vi "encoders_periodic.vi"() -> ()   [LabVIEW 2020]
uses:
  <vilib>/Rock Robotics/WPI/ThirdParty/Phoenix-LabVIEW/CANCoder/Get/CTRE_Phoenix_CANcoder_GetSensorData.vi
  Swerve/swerve_globals.vi
  <vilib>/Rock Robotics/WPI/ThirdParty/Phoenix-LabVIEW/CANCoder/Set/CTRE_Phoenix_CANcoder_SetPositionToAbsolute.vi
  TitanLib/Lib/TitanLib.lvlib
panel:
  in  "Set Mag Offset?":bool
  in  "Encoder Offsets":dbl[](array[numeric])
  out "Encoders":dbl[](array[numeric])
  in  "Reset Encoders?":bool
  # "Pos"
  # "Abs"
  # "Pos"
  # "Abs"
  # "Pos"
  # "Abs"
  # "Pos"
  # "Abs"
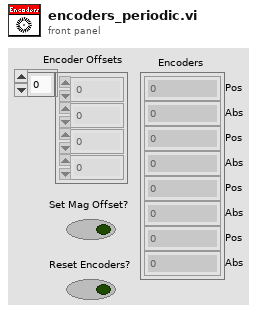
[diagram p1: front panel]
types:
  T1 = typedef "CTRE_Phoenix_CANcoder_DeviceRef.ctl" = cluster{"DeviceStatus":errorcluster, "Device Number":u8, "Handle":u64, "UsageFrame":u32, "Library Path":path}
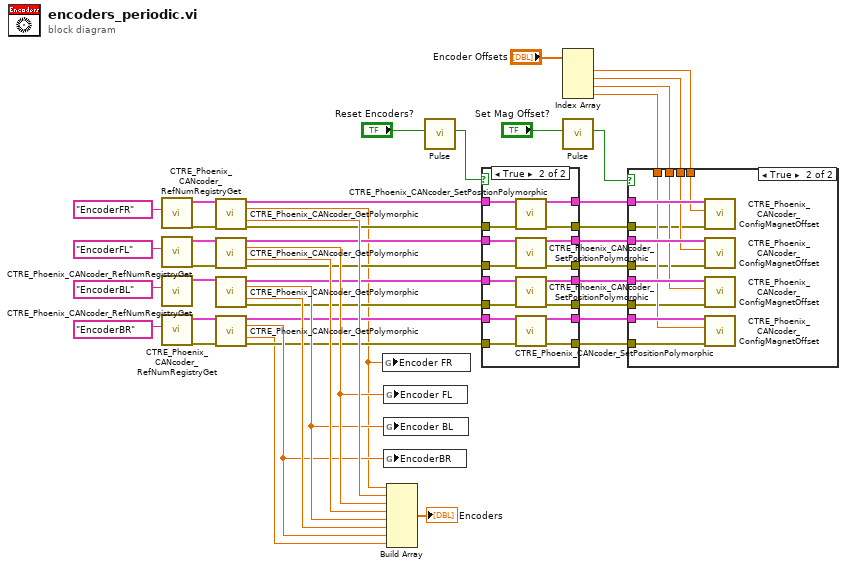
[diagram p0: block diagram]
diagram:
  n1 = call <vilib>:"CTRE_Phoenix_CANcoder_RefNumRegistryGet.vi"("refnum name"="EncoderFR") -> ("error out"=w11:errorcluster, "CTRE_CANcoder_DeviceRef"=w12:T1)  [unwired: 9 in]
  n2 = call <vilib>:"CTRE_Phoenix_CANcoder_RefNumRegistryGet.vi"("refnum name"="EncoderFL") -> ("error out"=w9:errorcluster, "CTRE_CANcoder_DeviceRef"=w10:T1)  [unwired: 9 in]
  n3 = call <vilib>:"CTRE_Phoenix_CANcoder_RefNumRegistryGet.vi"("refnum name"="EncoderBL") -> ("CTRE_CANcoder_DeviceRef"=w8:T1)  [unwired: 9 in, 1 out]
  n4 = call <vilib>:"CTRE_Phoenix_CANcoder_RefNumRegistryGet.vi"("refnum name"="EncoderBR") -> ("error out"=w6:errorcluster, "CTRE_CANcoder_DeviceRef"=w7:T1)  [unwired: 9 in]
  n5 = call-poly <vilib>:"CTRE_Phoenix_CANcoder_GetPolymorphic.vi"("CTRE_CANcoder_DeviceRef"=w12, "error in"=w11) -> ("CTRE_CANcoder_DeviceRef"=w39:T1, "Position"=w17:dbl, "Absolute Position"=w45:dbl, "error out"=w38:errorcluster)  [unwired: 9 in, 1 out]
  n6 = call-poly <vilib>:"CTRE_Phoenix_CANcoder_GetPolymorphic.vi"("CTRE_CANcoder_DeviceRef"=w10, "error in"=w9) -> ("CTRE_CANcoder_DeviceRef"=w37:T1, "Position"=w44:dbl, "Absolute Position"=w43:dbl, "error out"=w36:errorcluster)  [unwired: 9 in, 1 out]
  n7 = call-poly <vilib>:"CTRE_Phoenix_CANcoder_GetPolymorphic.vi"("CTRE_CANcoder_DeviceRef"=w8) -> ("CTRE_CANcoder_DeviceRef"=w35:T1, "Position"=w42:dbl, "Absolute Position"=w41:dbl, "error out"=w34:errorcluster)  [unwired: 10 in, 1 out]
  n8 = call-poly <vilib>:"CTRE_Phoenix_CANcoder_GetPolymorphic.vi"("CTRE_CANcoder_DeviceRef"=w7, "error in"=w6) -> ("CTRE_CANcoder_DeviceRef"=w33:T1, "Position"=w40:dbl, "Absolute Position"=w18:dbl, "error out"=w32:errorcluster)  [unwired: 9 in, 1 out]
  n9 = global write "swerve_globals.vi" "Encoder FR"(w17) -> ()
  n10 = global write "swerve_globals.vi" "Encoder FL"(w44) -> ()
  n11 = global write "swerve_globals.vi" "Encoder BL"(w42) -> ()
  n12 = global write "swerve_globals.vi" "EncoderBR"(w40) -> ()
  n13 = Build Array(w17, w45, w44, w43, w42, w41, w40, w18) -> (→"Encoders":dbl[])
  n14 = call "Pulse.vi"("Input"="Reset Encoders?") -> ("Output"=w30:bool)  [unwired: 10 in]
  n15 = case shown="True" w30 {
    tunnel: w39 -> [w53 w69]
    tunnel: w38 -> [w49 w68]
    tunnel: w37 -> [w52 w67]
    tunnel: w36 -> [w47 w66]
    tunnel: w35 -> [w51 w65]
    tunnel: w34 -> [w46 w64]
    tunnel: w33 -> [w50 w63]
    tunnel: w32 -> [w48 w62]
    tunnel: [w53 w61] -> w28
    tunnel: [w52 w60] -> w27
    tunnel: [w51 w59] -> w26
    tunnel: [w50 w58] -> w25
    tunnel: [w49 w56] -> w5
    tunnel: [w48 w57] -> w4
    tunnel: [w46 w55] -> w3
    tunnel: [w47 w54] -> w2
    frame False {
    }
    frame True {
      n16 = call-poly <vilib>:"CTRE_Phoenix_CANcoder_SetPositionPolymorphic.vi"("error in (no error)"=w68, "CTRE_CANcoder_DeviceRef"=w69) -> ("error out"=w56:errorcluster, "CTRE_CANcoder_DeviceRef"=w61:T1)  [unwired: 8 in]
      n17 = call-poly <vilib>:"CTRE_Phoenix_CANcoder_SetPositionPolymorphic.vi"("error in (no error)"=w66, "CTRE_CANcoder_DeviceRef"=w67) -> ("error out"=w54:errorcluster, "CTRE_CANcoder_DeviceRef"=w60:T1)  [unwired: 8 in]
      n18 = call-poly <vilib>:"CTRE_Phoenix_CANcoder_SetPositionPolymorphic.vi"("error in (no error)"=w64, "CTRE_CANcoder_DeviceRef"=w65) -> ("error out"=w55:errorcluster, "CTRE_CANcoder_DeviceRef"=w59:T1)  [unwired: 8 in]
      n19 = call-poly <vilib>:"CTRE_Phoenix_CANcoder_SetPositionPolymorphic.vi"("error in (no error)"=w62, "CTRE_CANcoder_DeviceRef"=w63) -> ("error out"=w57:errorcluster, "CTRE_CANcoder_DeviceRef"=w58:T1)  [unwired: 8 in]
    }
  }
  n20 = Index Array(array="Encoder Offsets") -> (element #1=w24:dbl, element #2=w23:dbl, element #3=w22:dbl, element #4=w21:dbl)  [unwired: 4 in]
  n21 = call "Pulse.vi"("Input"="Set Mag Offset?") -> ("Output"=w1:bool)  [unwired: 10 in]
  n22 = case shown="True" w1 {
    tunnel: w28 -> [_ w81]
    tunnel: w27 -> [_ w80]
    tunnel: w26 -> [_ w79]
    tunnel: w25 -> [_ w78]
    tunnel: w24 -> [_ w77]
    tunnel: w23 -> [_ w74]
    tunnel: w22 -> [_ w76]
    tunnel: w21 -> [_ w75]
    tunnel: w5 -> [_ w73]
    tunnel: w4 -> [_ w72]
    tunnel: w3 -> [_ w71]
    tunnel: w2 -> [_ w70]
    frame False {
    }
    frame True {
      n23 = call <vilib>:"CTRE_Phoenix_CANcoder_ConfigMagnetOffset.vi"("error in"=w73, "Magnet Offset (Degrees)"=w77, "CTRE_CANcoder_DeviceRef"=w81) -> ()  [unwired: 7 in, 2 out]
      n24 = call <vilib>:"CTRE_Phoenix_CANcoder_ConfigMagnetOffset.vi"("error in"=w70, "Magnet Offset (Degrees)"=w74, "CTRE_CANcoder_DeviceRef"=w80) -> ()  [unwired: 7 in, 2 out]
      n25 = call <vilib>:"CTRE_Phoenix_CANcoder_ConfigMagnetOffset.vi"("error in"=w71, "Magnet Offset (Degrees)"=w76, "CTRE_CANcoder_DeviceRef"=w79) -> ()  [unwired: 7 in, 2 out]
      n26 = call <vilib>:"CTRE_Phoenix_CANcoder_ConfigMagnetOffset.vi"("error in"=w72, "Magnet Offset (Degrees)"=w75, "CTRE_CANcoder_DeviceRef"=w78) -> ()  [unwired: 7 in, 2 out]
    }
  }
